vi "predict_extinction.vi"(8 "Error In":errorcluster, 11 "Xtal Description":T1) -> (0 "Error Out":errorcluster, 3 "prediction":dbl)   [LabVIEW 2019]
uses:
  xtal_description_for_prediction_cluster_typedef.ctl
panel:
  # "All inputs/outputs in radians!"
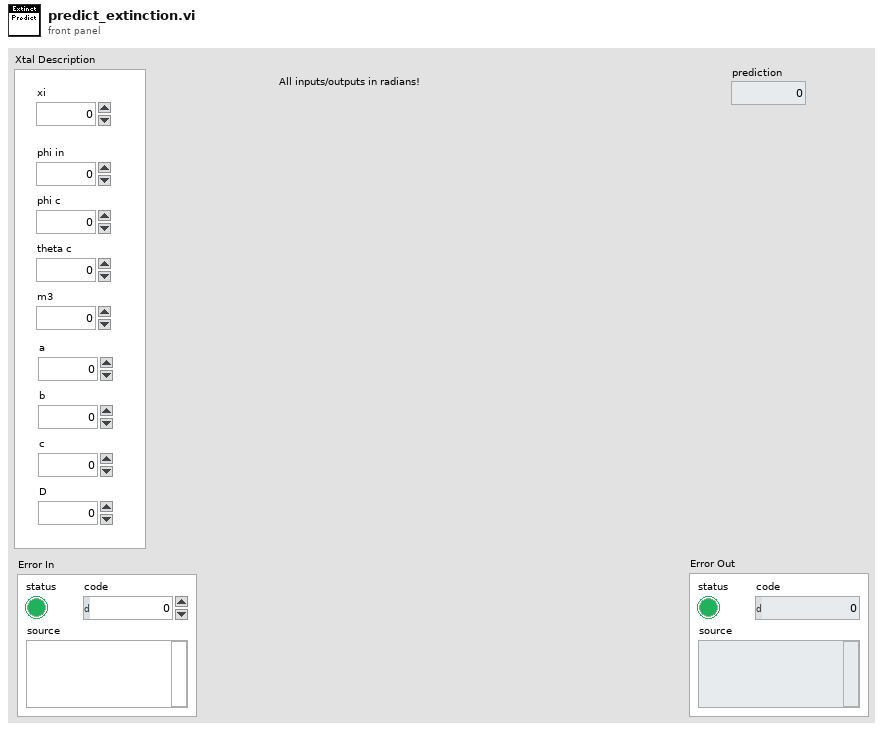
[diagram p1: front panel]
types:
  T1 = typedef "xtal_description_for_prediction_cluster_typedef.ctl" = cluster{"xi":dbl, "phi in":dbl, "phi c":dbl, "theta c":dbl, "m3":dbl, "a":dbl, "b":dbl, "c":dbl, "D":dbl}
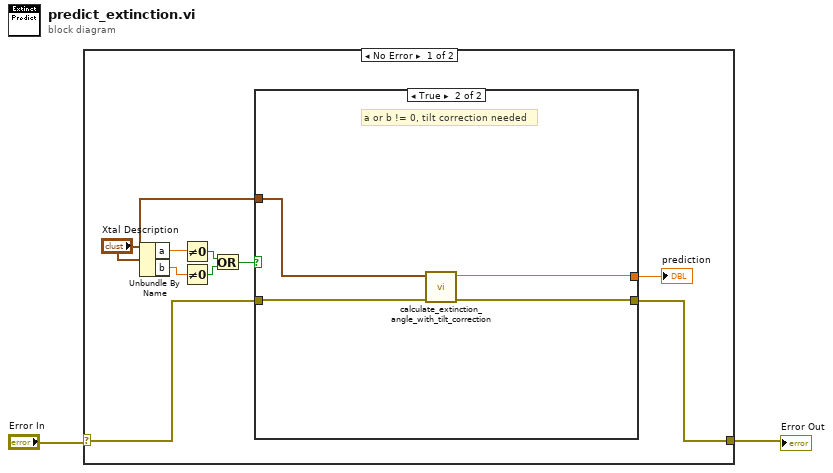
[diagram p0: block diagram]
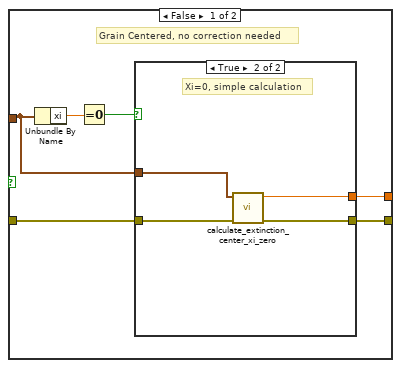
[diagram p2: hidden frame]
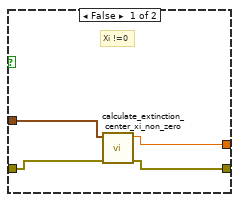
[diagram p3: hidden frame]
diagram:
  n1 = case shown="No Error" "Error In" {
    selector: "Error In" -> [w3 w30]
    tunnel: [w4 w30] -> w1
    frame No Error {
      n2 = Unbundle By Name("Xtal Description") -> ("a"=w11:dbl, "b"=w10:dbl)
      n3 = Not Equal To 0?(x=w11) -> (x != 0?=w9:bool)
      n4 = Not Equal To 0?(x=w10) -> (x != 0?=w8:bool)
      n5 = Or(x=w9, y=w8) -> (x .or. y?=w7:bool)
      n6 = case shown="True" w7 {
        tunnel: "Xtal Description" -> [w12 w26]
        tunnel: [w15 w29] -> w5
        tunnel: [w14 w28] -> w4
        tunnel: w3 -> [w13 w27]
        frame False {
          # "Grain Centered, no correction needed"
          n7 = Unbundle By Name(w12) -> ("xi"=w17:dbl)
          n8 = Equal To 0?(x=w17) -> (x = 0?=w16:bool)
          n9 = case shown="True" w16 {
            tunnel: [w18 w25] -> w15
            tunnel: [w19 w24] -> w14
            tunnel: w13 -> [w20 w23]
            tunnel: w12 -> [w21 w22]
            frame False {
              # "Xi !=0"
              n10 = call "calculate_extinction_center_xi_non_zero.vi"("Error In"=w20, "Xtal Description"=w21) -> ("Error Out"=w19:errorcluster, "prediction"=w18:dbl)  [unwired: 8 in]
            }
            frame True {
              # "Xi=0, simple calculation"
              n11 = call "calculate_extinction_center_xi_zero.vi"("Error In"=w23, "Xtal Description"=w22) -> ("Error Out"=w24:errorcluster, "prediction"=w25:dbl)  [unwired: 8 in]
            }
          }
        }
        frame True {
          # "a or b != 0, tilt correction needed"
          n12 = call "calculate_extinction_angle_with_tilt_correction.vi"("Error In"=w27, "Xtal Description"=w26) -> ("Error Out"=w28:errorcluster, "prediction"=w29:dbl)  [unwired: 8 in]
        }
      }
      "prediction" <- w5
    }
    frame Error {
    }
  }
  "Error Out" <- w1
